vi "SendFirmware.vi"(8 "Error in":errorcluster, 9 "Progress notifier":refnum<notifier>, 10 "Data In":u32[](array[numeric]), 11 "Channel In":u16) -> (0 "Error out":errorcluster, 3 "Channel Out":u16)   [LabVIEW 2022 SP3]
uses:
  Program Files/National Instruments/LabVIEW 2024/user.lib/pcanbasic/PCANBasic.lvlib
panel:
  out "Numeric":i32
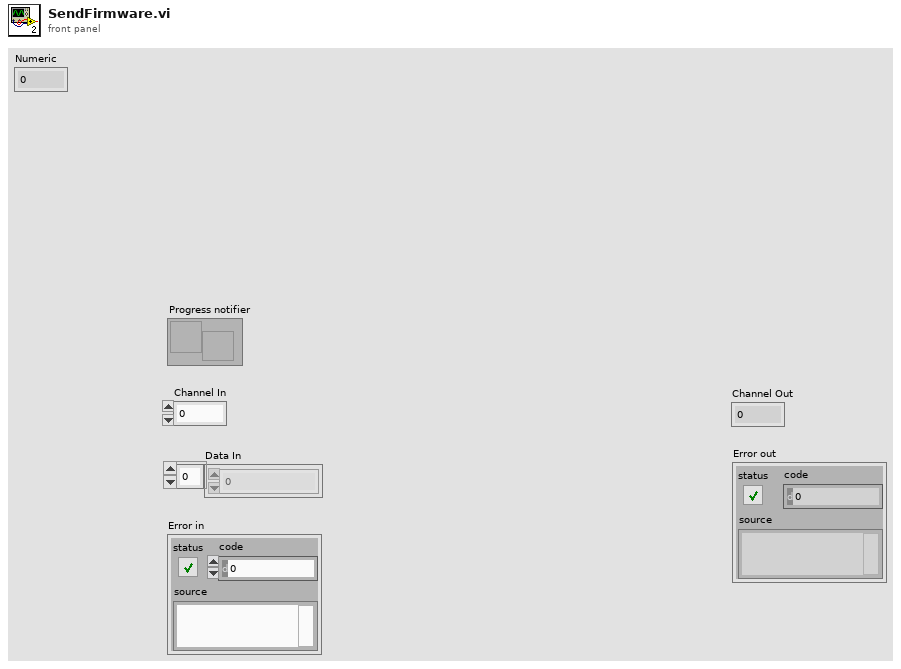
[diagram p1: front panel]
types:
  T1 = cluster{"ID":u32, "MSGTYPE":u8, "LEN":u8, "DATA[0]":u8, "DATA[1]":u8, "DATA[2]":u8, "DATA[3]":u8, "DATA[4]":u8, "DATA[5]":u8, "DATA[6]":u8, "DATA[7]":u8}
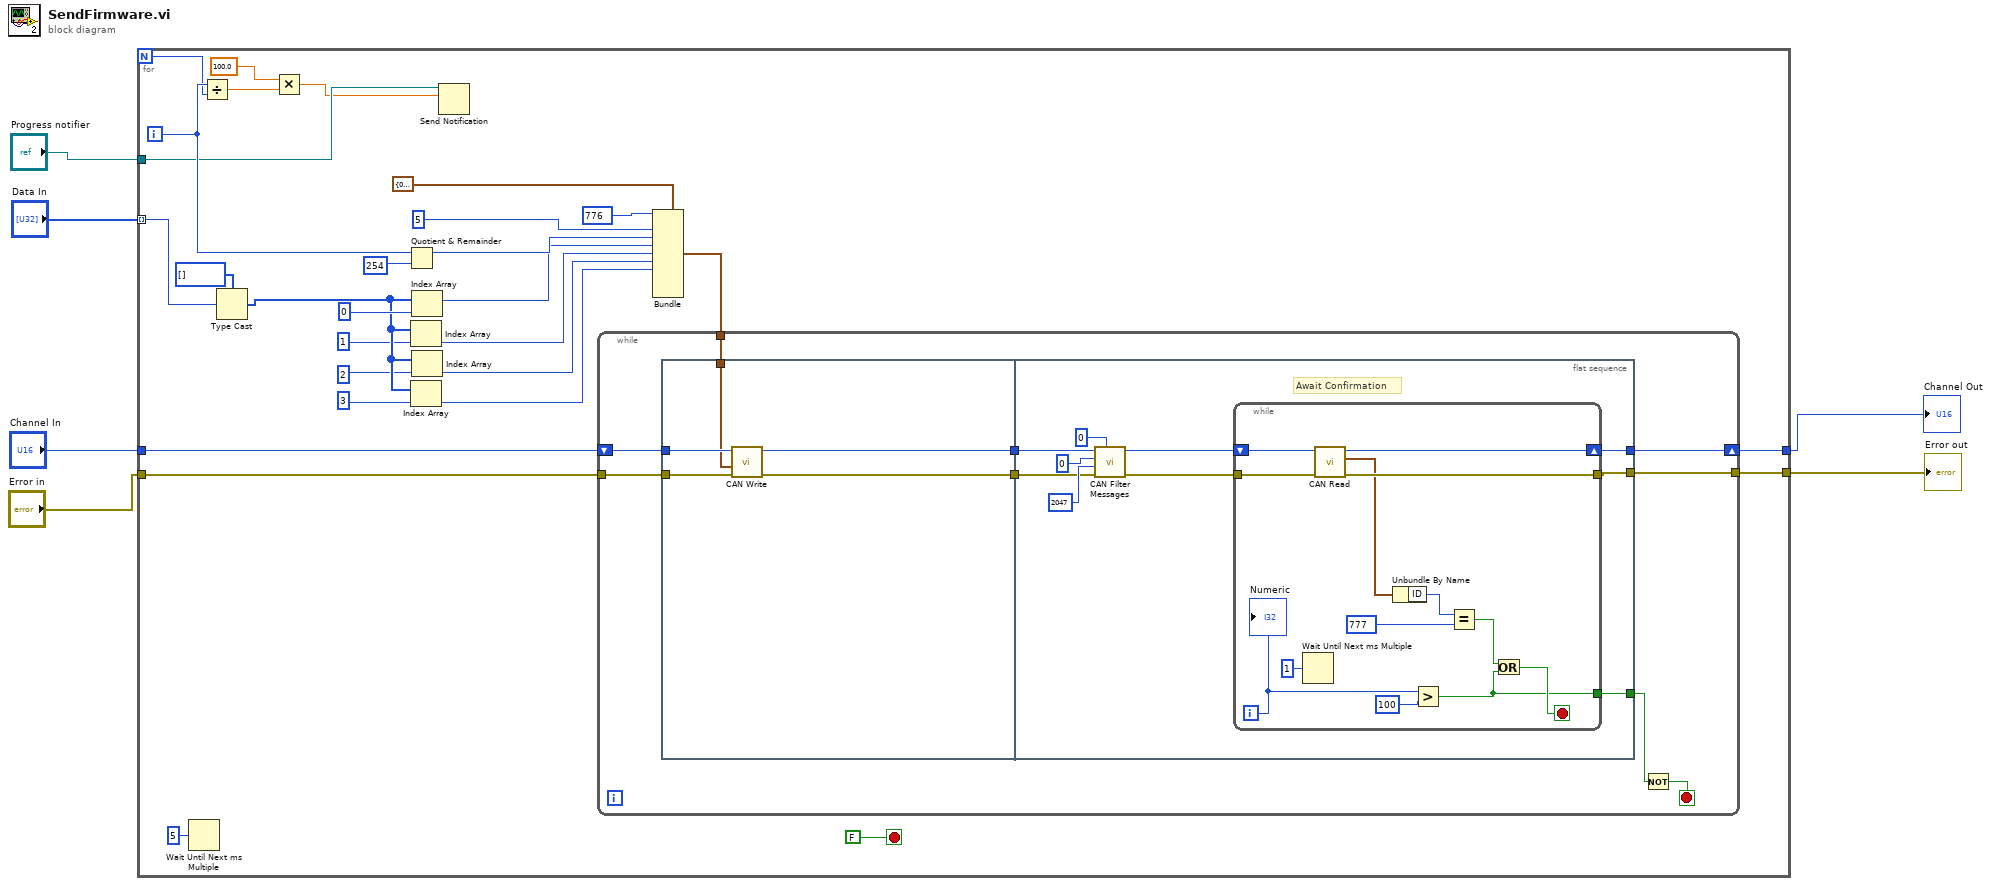
[diagram p0: block diagram]
diagram:
  n1 = for {
    N -> [w11]
    tunnel: "Data In" -> [w26] mode=indexing
    tunnel: "Channel In" -> [w33]
    tunnel: "Error in" -> [w28]
    tunnel: [w19] -> w2
    tunnel: [w9] -> w3
    tunnel: "Progress notifier" -> [w8]
    i -> [w12]
    stop <- FALSE stop-if-true
    n2 = Wait Until Next ms Multiple(millisecond multiple=u32 5) -> ()  [unwired: 1 out]
    n3 = Divide(x=w12, y=w11) -> (x/y=w35:dbl)
    n4 = Type Cast(type=u8[] [], x=w26) -> (*(type *) &x=w23:u8[])
    n5 = Multiply(x=100.0, y=w35) -> (x*y=w7:dbl)
    n6 = Quotient & Remainder(x=w12, y=254) -> (x-y*floor(x/y)=w17:i32)  [unwired: 1 out]
    n7 = Index Array(array=w23, index=1) -> (element=w15:u8)
    n8 = Index Array(array=w23, index=3) -> (element=w13:u8)
    n9 = Index Array(array=w23, index=0) -> (element=w16:u8)
    n10 = Index Array(array=w23, index=2) -> (element=w14:u8)
    n11 = Send Notification(notification=w7, notifier=w8) -> ()  [unwired: 1 in, 2 out]
    n12 = Bundle(cluster=T1 {"ID"=0, "MSGTYPE"=0, "LEN"=0, "DATA[0]"=0, "DATA[1]"=0, "DATA[2]"=0, "DATA[3]"=0, "DATA[4]"=0, "DATA[5]"=0, "DATA[6]"=0, "DATA[7]"=0} ("MessageBuffer"), "ID"=u32 776, "LEN"=u8 5, "DATA[0]"=w17, "DATA[1]"=w16, "DATA[2]"=w15, "DATA[3]"=w14, "DATA[4]"=w13) -> (w29:T1)  [unwired: 4 in]
    n13 = while {
      tunnel: w29 -> [w41]
      tunnel: w28 -> [w40]
      shift-right: [w39] -> w19
      shift-left: w33 -> [w42]
      tunnel: [w36] -> w9
      stop <- w37 stop-if-true
      n14 = flat-sequence {
        tunnel: w42 -> [w49]
        tunnel: w41 -> [w48]
        tunnel: w40 -> [w47]
        tunnel: [w46] -> w44
        tunnel: [w45] -> w43
        tunnel: [w59] -> w39
        tunnel: w44 -> [w55]
        tunnel: w43 -> [w53]
        tunnel: [w51] -> w38
        tunnel: [w50] -> w36
        frame #0 {
          n15 = call "CAN Write.vi"("error in (no error)"=w47, "MessageBuffer"=w48, "Channel"=w49) -> ("error out"=w45:errorcluster, "Channel Out"=w46:u16)  [unwired: 5 in, 2 out]
        }
        frame #1 {
          # "Await Confirmation"
          n16 = call "CAN Filter Messages.vi"("Mode"=u8 0, "error in (no error)"=w53, "ToID"=u32 2047, "FromID"=u32 0, "Channel"=w55) -> ("error out"=w52:errorcluster, "Channel Out"=w54:u16)  [unwired: 4 in, 1 out]
          n17 = while {
            shift-right: [w72] -> w59
            shift-left: w54 -> [w71]
            tunnel: w52 -> [w70]
            tunnel: [w69] -> w50
            tunnel: [w60] -> w51
            i -> [w64]
            stop <- w61 stop-if-true
            n18 = Wait Until Next ms Multiple(millisecond multiple=u32 1) -> ()  [unwired: 1 out]
            n19 = call "CAN Read.vi"("error in (no error)"=w70, "Channel"=w71) -> ("error out"=w69:errorcluster, "MessageBuffer out"=w67:T1, "Channel Out"=w72:u16)  [unwired: 5 in, 2 out]
            n20 = Unbundle By Name(w67) -> ("ID"=w66:u32)
            n21 = Greater?(x=w64, y=100) -> (0:w60:bool)
            n22 = Equal?(x=w66, y=u32 777) -> (x = y?=w62:bool)
            n23 = Or(x=w62, y=w60) -> (x .or. y?=w61:bool)
            "Numeric" <- w64
          }
        }
      }
      n24 = Not(x=w38) -> (.not. x?=w37:bool)
    }
  }
  "Error out" <- w3
  "Channel Out" <- w2
